vi "Send.vi"(8 "error in (no error)":errorcluster, 10 "Command":string, 11 "EPU452 in":refnum<class "EPU452.lvclass">) -> (0 "error out":errorcluster, 3 "EPU452 out":refnum<class "EPU452.lvclass">)   [LabVIEW 2018, in "EPU452.lvclass"]
uses:
  EPU452.lvclass
  EPU452.lvclass/EPU452.ctl
  <vilib>/Instr/_visa.llb/VISA Flush IO Buffer Mask.ctl
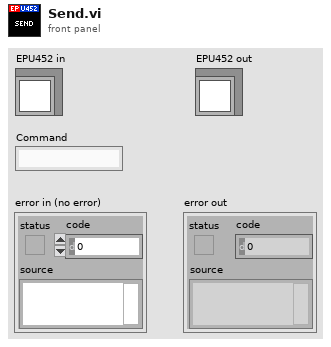
[diagram p1: front panel]
types:
  T1 = typedef "VISA Flush IO Buffer Mask.ctl" = u16
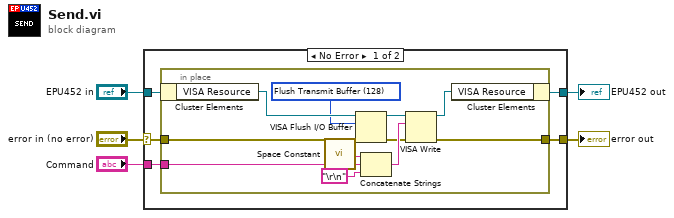
[diagram p0: block diagram]
diagram:
  n1 = case shown="No Error" "error in (no error)" {
    selector: "error in (no error)" -> [w10 w23]
    tunnel: [w9 w23] -> w4
    tunnel: [w6 w22] -> w2
    tunnel: "EPU452 in" -> [w8 w22]
    tunnel: "Command" -> [w7 _]
    frame No Error {
      n2 = in-place {
        in-place-border: w10 -> [w15]
        in-place-border: [w17] -> w9
        in-place-border: w7 -> [w19]
        w11 = T1 128 items=["Flush Receive Buffer"=16, "Write Transmit Buffer to Device"=32, "Flush Receive Buffer (No I/O)"=64, "Flush Transmit Buffer"=128] ("Mask")
        n3 = in-place-cluster #1(w8) -> ("VISA Resource"=w13:refnum<visa-resource-name>)
        n4 = call <vilib>:"Space Constant.vi"() -> ("String"=w18:string)
        n5 = VISA Flush I/O Buffer(VISA resource name=w13, mask (16)=w11, error in (no error)=w15) -> (VISA resource name out=w12:refnum<visa-resource-name>, error out=w14:errorcluster)
        n6 = Concatenate Strings(w18, w19, "\r\n") -> (w20:string)
        n7 = VISA Write(VISA resource name=w12, write buffer=w20, error in (no error)=w14) -> (VISA resource name out=w16:refnum<visa-resource-name>, error out=w17:errorcluster)  [unwired: 1 out]
        n8 = in-place-cluster #1("VISA Resource"=w16) -> (w6:refnum<class "EPU452.lvclass">)
      }
    }
    frame Error {
    }
  }
  "error out" <- w4
  "EPU452 out" <- w2
